vi "Color Sensor V3 Color Match FGV.vi"(10 "Get Only? (F)":bool, 11 "Color Match":T1) -> (3 "All Match Colors":T1[](array[typedef]))   [LabVIEW 2019]
uses:
  TypeDef/Color Sensor V3 Color Match.ctl
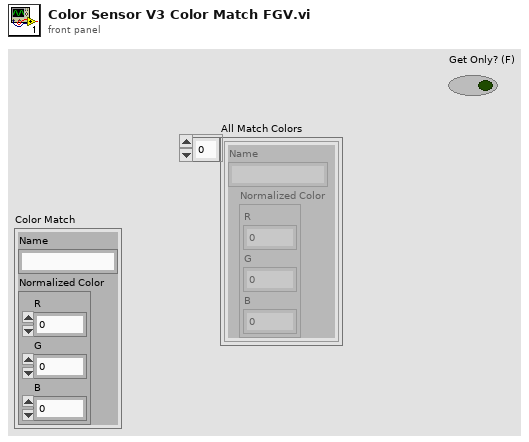
[diagram p1: front panel]
types:
  T1 = typedef "Color Sensor V3 Color Match.ctl" = cluster{"Name":string, "Normalized Color":cluster{"R":dbl, "G":dbl, "B":dbl}}
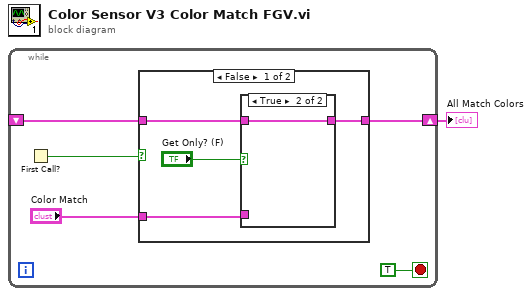
[diagram p0: block diagram]
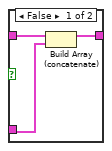
[diagram p2: hidden frame]
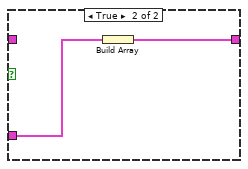
[diagram p3: hidden frame]
diagram:
  n1 = while {
    shift-right: [w4] -> w1
    shift-left: _ -> [w3]
    stop <- TRUE stop-if-true
    n2 = First Call?() -> (First Call?: T/F=w5:bool)
    n3 = case shown="False" w5 {
      tunnel: "Color Match" -> [w10 w16]
      tunnel: [w8 w15] -> w4
      tunnel: w3 -> [w9 _]
      frame False {
        n4 = case shown="True" "Get Only? (F)" {
          tunnel: w10 -> [w13 _]
          tunnel: w9 -> [w12 w14]
          tunnel: [w11 w14] -> w8
          frame False {
            n5 = Build Array (concatenate)(w12, w13) -> (w11:T1[])
          }
          frame True {
          }
        }
      }
      frame True {
        n6 = Build Array(w16) -> (w15:T1[])
      }
    }
  }
  "All Match Colors" <- w1
